vi "Edit Plugin Type Specialization - Multiple Converter.vi"(11 "error in":errorcluster) -> (15 "error out":errorcluster)   [LabVIEW 2021, in "Converter.lvlib"]
uses:
  Converter.lvlib
  Path Functions/Path Functions.lvlib
  Converter Reusables/Converter Reusables.lvlib
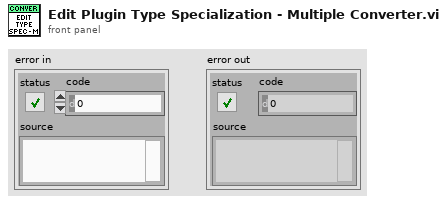
[diagram p1: front panel]
types:
  T1 = cluster{"parameter name":string, "type specialization":enum16{"none", "pin", "path", "enum"}, "annotations":cluster{"key":enum16{"none", "pin.instrument_type", "enum.values"}, "value":string}[]}[]
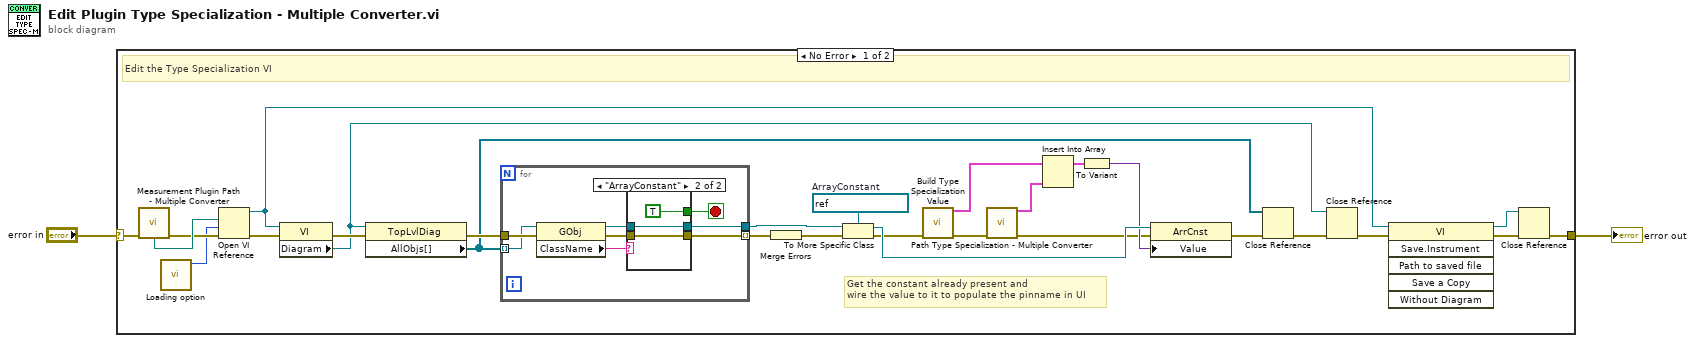
[diagram p0: block diagram]
diagram:
  n1 = case shown="No Error" "error in" {
    selector: "error in" -> [w10 w43]
    tunnel: [w5 w43] -> w1
    frame No Error {
      w22 = refnum<vi> refnum  # ArrayConstant
      # "Get the constant already present and\nwire the value to it to populate the pinname in UI"
      # "Edit the Type Specialization VI"
      n2 = call "Measurement Plugin Path - Multiple Converter.vi"("error in"=w10) -> ("type specialization"=w11:path, "error out"=w9:errorcluster)  [unwired: 2 in, 11 out]
      n3 = call "Loading option.vi"() -> ("options"=w3:i32)  [unwired: 11 in]
      n4 = Open VI Reference(vi path=w11, options=w3, error in (no error)=w9) -> (vi reference=w18:refnum<vi>, error out=w30:errorcluster)  [unwired: 3 in]
      n5 = property class="VI"(reference=w18, error in=w30) -> (error out=w29:errorcluster, "Diagram"=w24:refnum<vi>)  [unwired: 1 out]
      n6 = property class="TopLvlDiag"(reference=w24, error in=w29) -> (error out=w28:errorcluster, "AllObjs[]"=w25:refnum<vi>[])  [unwired: 1 out]
      n7 = for {
        tunnel: w25 -> [w37] mode=indexing
        tunnel: w28 -> [w38]
        tunnel: [w34] -> w23
        tunnel: [w32] -> w21 mode=indexing
        stop <- w33 stop-if-true
        n8 = property class="GObj"(reference=w37, error in=w38) -> (reference out=w35:refnum<vi>, error out=w36:errorcluster, "ClassName"=w31:string)
        n9 = case shown="\"ArrayConstant\"" w31 {
          tunnel: w36 -> [w39 w41]
          tunnel: w35 -> [_ w42]
          tunnel: [_ w42] -> w34
          tunnel: [_ TRUE] -> w33
          tunnel: [w39 w41] -> w32
          frame Default {
          }
          frame "ArrayConstant" {
          }
        }
      }
      n10 = Merge Errors(w21) -> (w20:errorcluster)
      n11 = To More Specific Class(target class=w22, reference=w23, error in=w20) -> (specific class reference=w17:refnum<vi>, error out=w16:errorcluster)
      n12 = call "Build Type Specialization Value.vi"("error in"=w16) -> ("type specialization"=w13:T1, "error out"=w7:errorcluster)  [unwired: 13 in]
      n13 = call "Path Type Specialization - Multiple Converter.vi"("error in"=w7) -> ("type specialization for path"=w8:T1, "error out"=w6:errorcluster)  [unwired: 13 in]
      n14 = Insert Into Array(array=w13, new element=w8) -> (w12:T1)  [unwired: 1 in]
      n15 = To Variant(anything=w12) -> (Variant=w15:variant)
      n16 = property class="ArrCnst"(reference=w17, error in=w6, "Value"=w15) -> (error out=w4:errorcluster)  [unwired: 1 out]
      n17 = Close Reference(reference=w25, error in (no error)=w4) -> (error out=w27:errorcluster)
      n18 = Close Reference(reference=w24, error in (no error)=w27) -> (error out=w26:errorcluster)
      n19 = invoke class="VI" method="Save.Instrument"(reference=w18, error in=w26) -> (reference out=w14:refnum<vi>, error out=w19:errorcluster)  [unwired: 4 in, 4 out]
      n20 = Close Reference(reference=w14, error in (no error)=w19) -> (error out=w5:errorcluster)
    }
    frame Error {
    }
  }
  "error out" <- w1
